vi "NetComm_getAllianceStation.vi"(8 "error in (no error)":errorcluster) -> (0 "error out":errorcluster, 2 "Alliance Station":T1)   [LabVIEW 2017]
uses:
  <vilib>/Rock Robotics/SystemInterfaces/NetworkCommunication/NetComm_AllianceStation.ctl
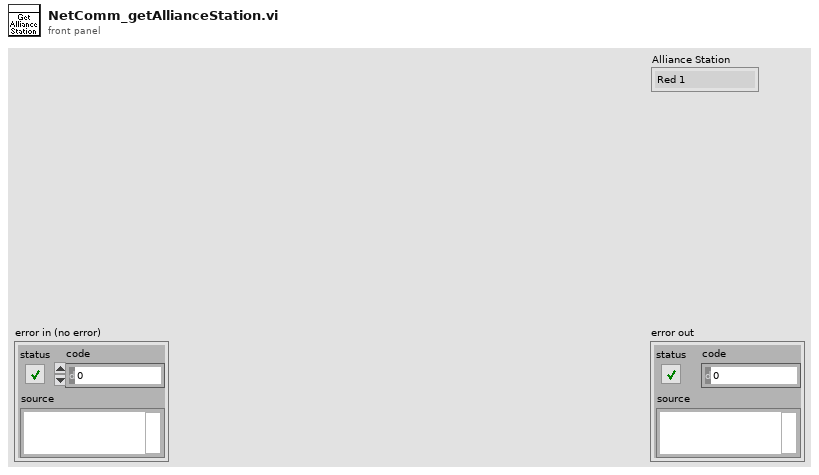
[diagram p1: front panel]
types:
  T1 = typedef "NetComm_AllianceStation.ctl" = enum16{"Red 1", "Red 2", "Red 3", "Blue 1", "Blue 2", "Blue 3"}
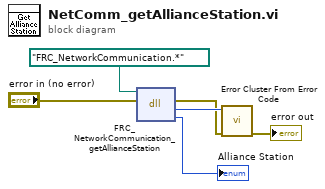
[diagram p0: block diagram]
diagram:
  n1 = dll-call lib="?" fn="FRC_NetworkCommunication_getAllianceStation"(path in=path "FRC_NetworkCommunication.*", error in="error in (no error)") -> (error out=w3:errorcluster, "return type"=w5:i32, "allianceStation"=→"Alliance Station":i32)  [unwired: 2 in, 1 out]
  n2 = call <vilib>:"Error Cluster From Error Code.vi"("error in (no error)"=w3, "error code (0)"=w5) -> ("error out"=→"error out":errorcluster)  [unwired: 7 in]
